vi "FindTargetCtlReference.vi"(8 "error in (no error)":errorcluster, 10 "TargetCtlLabel.Text":string, 11 "AllControlReference":refnum<vi>[](array[refnum])) -> (0 "error out":errorcluster, 2 "Find?":bool, 3 "TargetCtlRefnum":refnum<vi>)   [LabVIEW 2013]
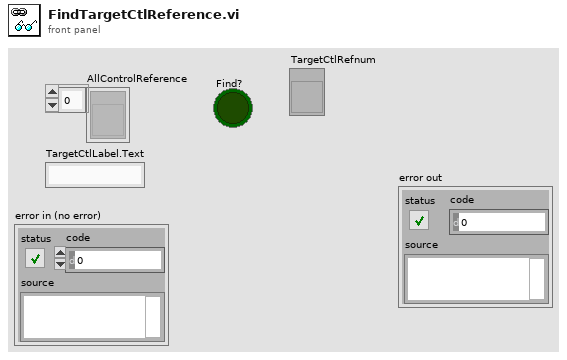
[diagram p1: front panel]
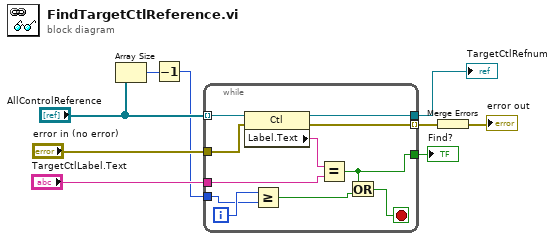
[diagram p0: block diagram]
diagram:
  n1 = Array Size(array="AllControlReference") -> (size(s)=w3:i32)
  n2 = Decrement(x=w3) -> (x-1=w2:i32)
  n3 = while {
    tunnel: "AllControlReference" -> [w20] mode=indexing
    tunnel: "TargetCtlLabel.Text" -> [w19]
    tunnel: [w17] -> w7
    tunnel: "error in (no error)" -> [w16]
    tunnel: [w15] -> w4 mode=indexing
    tunnel: [w12] -> w6
    tunnel: w2 -> [w13]
    i -> [w14]
    stop <- w10 stop-if-true
    n4 = property class="Ctl"(reference=w20, error in=w16) -> (reference out=w17:refnum<vi>, error out=w15:errorcluster, "Label.Text"=w18:string)
    n5 = Greater Or Equal?(x=w14, y=w13) -> (x >= y?=w11:bool)
    n6 = Equal?(x=w18, y=w19) -> (x = y?=w12:bool)
    n7 = Or(x=w12, y=w11) -> (x .or. y?=w10:bool)
  }
  "TargetCtlRefnum" <- w7
  "Find?" <- w6
  n8 = Merge Errors(w4) -> (→"error out":errorcluster)
